vi "DeBounce.vi"(10 "DB_Count":dbl, 11 "Value":bool) -> (3 "BD_Value":bool)   [LabVIEW 2015]
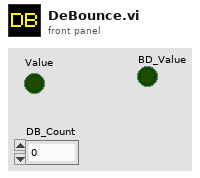
[diagram p1: front panel]
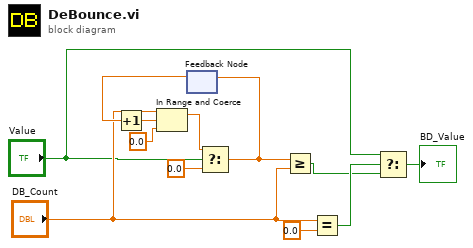
[diagram p0: block diagram]
diagram:
  n1 = feedback #1() -> (w10:dbl)  [unwired: 1 in]
  n2 = Increment(x=w10) -> (x+1=w9:dbl)
  n3 = In Range and Coerce(upper limit="DB_Count", x=w9, lower limit=0.0) -> (coerced(x)=w7:dbl)  [unwired: 1 out]
  n4 = Select(t=w7, s="Value", f=0.0) -> (s? t:f=w11:dbl)
  n5 = feedback-in #1(w11) -> ()
  n6 = Greater Or Equal?(x=w11, y="DB_Count") -> (x >= y?=w2:bool)
  n7 = Equal?(x="DB_Count", y=0.0) -> (x = y?=w4:bool)
  n8 = Select(t="Value", s=w4, f=w2) -> (s? t:f=→"BD_Value":bool)
